vi "can_event.vi"() -> ()   [LabVIEW 2009]
doc: "This example demonstrates the use of Local Variables with Boolean controls. It uses a typical parallel loop architecture; in order to stop both loops at the same time it uses a local variable to read the switch value.\n\nThe example simulates the \"latch when pressed\" mechanical action by using another local variable to reset the switch to the FALSE value. This is needed because the actual \"latch when pressed\" mechanical action is not compatible with local variables.\n\nRefer to the \"Stopping Parallel While Loops without Reset\" example for a demonstration of what would happen if the switch was not reset."
panel:
  out "Write Error out":errorcluster {"code" format="%.0x"}
  out "Read Error out":errorcluster {"code" format="%.0x"}
  out "send status":bool
  out "receive status":bool
  out "Received MSG":string[][](table)
  in  "Receive Data Format":enum32{"Hexadecimal", "Decimal"}(radio)
  in  "MSG_RTR":bool
  in  "Flags":u8(ring)=4 items=["MSG_STD"=0, "MSG_EXT"=4]
  in  "ID (HEX)":u32=2047 format="%x"
  in  "Number to Write":u32=100
  out "Transmission MSG":string[][](table)
  in  "Write Data Format":enum32{"Hexadecimal", "Decimal"}(radio)
  in  "Read CANPort":string(combo)="CAN1"
  in  "Write CANPort":string(combo)="CAN2"
  out "GetEventMask":u32(ring)=129 items=["EV_ERR+EV_RXCHAR"=129]
  in  "ReadCount":u32=100
  out "WaitEvent\nErrorCode":u32
  in  "stop":bool
  out "Write Overlapped":T1
  out "Write Handle":u32
  out "Read Overlapped":T2
  out "Read Handle":u32
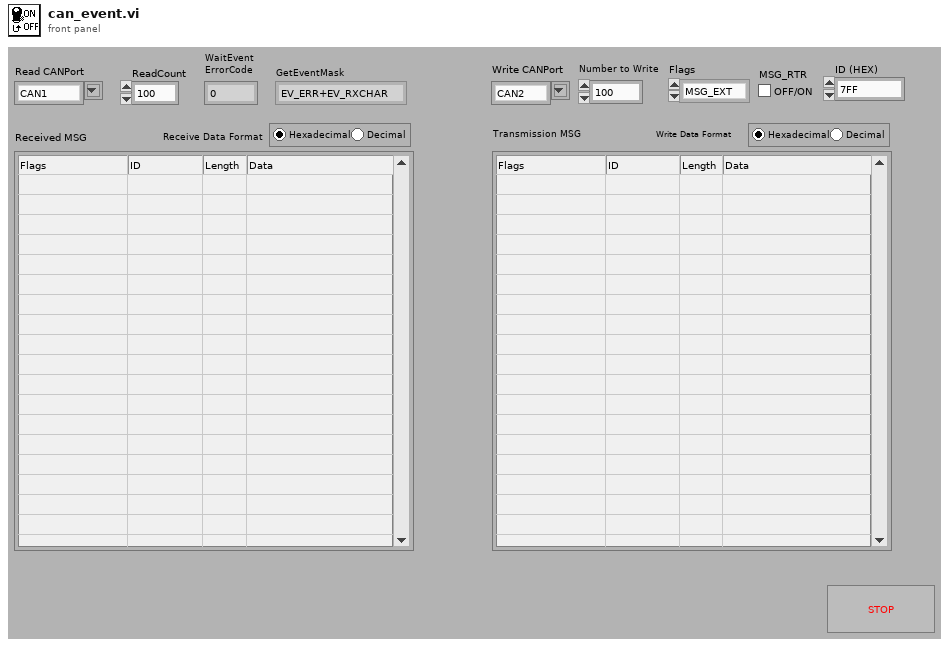
[diagram p1: front panel]
types:
  T1 = cluster{"Internal":u32, "InternalHigh":u32, "Offset":u32, "OffsetHigh":u32, "hEvent":u32}
  T2 = cluster{"Numeric":u32, "Numeric 2":u32, "Numeric 3":u32, "Numeric 4":u32, "Numeric 5":u32}
  T3 = cluster{"Flags":u32, "ID(HEX)":u32, "Length":i16, "Data":u8[]}[]
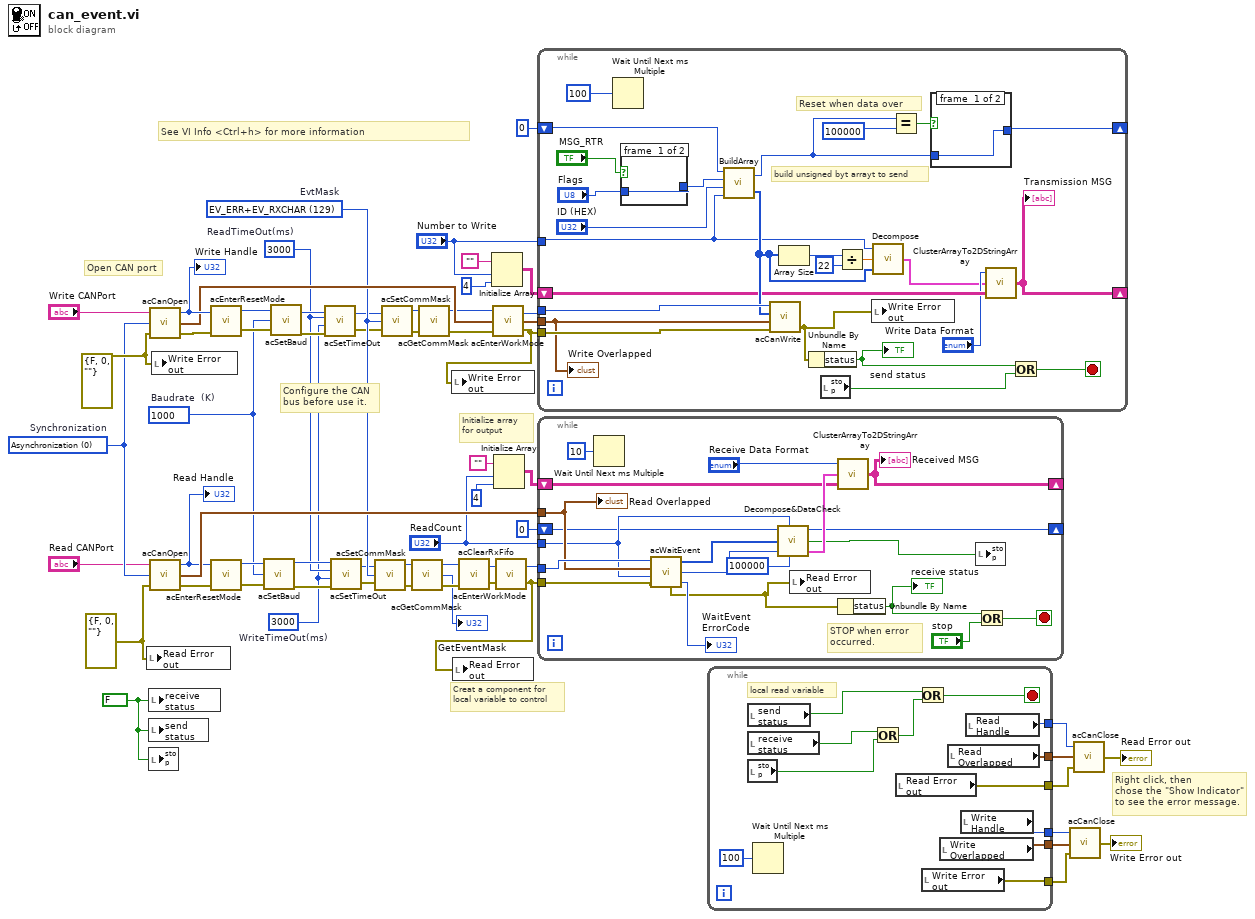
[diagram p0: block diagram]
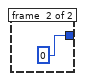
[diagram p2: hidden frame]
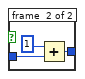
[diagram p3: hidden frame]
diagram:
  w1 = FALSE ("receive status")
  w20 = u32 3000  # WriteTimeOut(ms)
  w21 = u32 3000  # ReadTimeOut(ms)
  w19 = u16 1000 items=["10"=10, "20"=20, "50"=50, "100"=100, "125"=125, "250"=250, "500"=500, "800"=800, "1000"=1000]  # Baudrate  (K)
  w44 = 0 items=["Synchronization"=1, "Asynchronization"=0]  # Synchronization
  w45 = errorcluster {"status"=FALSE, "code"=0, "source"=""} ("Error in")
  w37 = u32 129 items=["EV_ERR+EV_RXCHAR"=129]  # EvtMask
  w54 = errorcluster {"status"=FALSE, "code"=0, "source"=""} ("Error in")
  # "Open CAN port"
  # "Creat a component for \nlocal variable to control"
  # "Configure the CAN \nbus before use it."
  # "See VI Info <Ctrl+h> for more information"
  # "Initialize array \nfor output"
  # "Right click, then \nchose the \"Show Indicator\" \nto see the error message."
  n1 = local write "Read Error out"(w54) -> ()
  n2 = local write "receive status"(w1) -> ()
  n3 = local write "send status"(w1) -> ()
  n4 = local write "stop"(w1) -> ()
  n5 = call "acCanOpen.vi"("Error in"=w45, "Synchronization"=w44, "CANPort"="Write CANPort") -> ("Error out"=w43:errorcluster, "Overlapped"=w40:T1, "Handle"=w42:u32)
  "Write Handle" <- w42
  n6 = call "acCanOpen.vi"("Error in"=w54, "Synchronization"=w44, "CANPort"="Read CANPort") -> ("Error out"=w33:errorcluster, "Overlapped"=w59:T1, "Handle"=w34:u32)
  "Read Handle" <- w34
  n7 = local write "Write Error out"(w45) -> ()
  n8 = call "acEnterResetMode.vi"("Error in"=w43, "Handle  in"=w42) -> ("Error out"=w32:errorcluster, "Handle out"=w18:u32)
  n9 = call "acEnterResetMode.vi"("Error in"=w33, "Handle  in"=w34) -> ("Error out"=w22:errorcluster, "Handle out"=w23:u32)
  n10 = call "acSetBaud.vi"("Error in"=w22, "Baudrate"=w19, "Handle  in"=w23) -> ("Error out"=w27:errorcluster, "Handle out"=w26:u32)
  n11 = call "acSetBaud.vi"("Error in"=w32, "Baudrate"=w19, "Handle  in"=w18) -> ("Error out"=w30:errorcluster, "Handle out"=w31:u32)
  n12 = call "acSetTimeOut.vi"("Error in"=w30, "WriteTimeOut"=w20, "Read TimeOut"=w21, "Handle  in"=w31) -> ("Error out"=w28:errorcluster, "Handle out"=w29:u32)
  n13 = call "acSetTimeOut.vi"("Error in"=w27, "WriteTimeOut"=w20, "Read TimeOut"=w21, "Handle  in"=w26) -> ("Error out"=w25:errorcluster, "Handle out"=w24:u32)
  n14 = call "acSetCommMask.vi"("Error in"=w25, "EventMask"=w37, "Handle  in"=w24) -> ("Error out"=w61:errorcluster, "Handle out"=w60:u32)  [unwired: 1 in]
  n15 = call "acSetCommMask.vi"("Error in"=w28, "EventMask"=w37, "Handle  in"=w29) -> ("Error out"=w39:errorcluster, "Handle out"=w38:u32)  [unwired: 1 in]
  n16 = call "acGetCommMask.vi"("Handle  in"=w60, "Error in"=w61) -> ("Handle out"=w46:u32, "GetEventMask"=→"GetEventMask":u32, "Error out"=w47:errorcluster)
  n17 = call "acGetCommMask.vi"("Handle  in"=w38, "Error in"=w39) -> ("Handle out"=w2:u32, "Error out"=w3:errorcluster)  [unwired: 1 out]
  n18 = call "acClearRxFifo.vi"("Error in"=w47, "Handle  in"=w46) -> ("Error out"=w49:errorcluster, "Handle out"=w48:u32)
  n19 = Initialize Array("", "Number to Write", 4 ("Dimension Size")) -> (w13:string[][])
  n20 = call "acEnterWorkMode.vi"("Error in"=w3, "Handle  in"=w2) -> ("Error out"=w4:errorcluster, "Handle out"=w41:u32)
  n21 = local write "Write Error out"(w4) -> ()
  n22 = Initialize Array("", "ReadCount", 4 ("Dimension Size")) -> (w8:string[][])
  n23 = call "acEnterWorkMode.vi"("Error in"=w49, "Handle  in"=w48) -> ("Error out"=w6:errorcluster, "Handle out"=w56:u32)
  n24 = local write "Read Error out"(w6) -> ()
  n25 = while {
    tunnel: w41 -> [w87]
    tunnel: w4 -> [w86]
    tunnel: w40 -> [w85]
    shift-right: [w66] -> _
    shift-left: 0 ("Numberto out") -> [w82]
    shift-right: [w75] -> _
    shift-left: w13 -> [w76]
    tunnel: "Number to Write" -> [w77]
    stop <- w62 stop-if-true
    # "Reset when data over"
    # "build unsigned byt arrayt to send"
    n26 = Wait Until Next ms Multiple(millisecond multiple=u32 100) -> ()  [unwired: 1 out]
    n27 = case shown="False" "MSG_RTR" {
      tunnel: "Flags" -> [w90 w93]
      tunnel: [w90 w91] -> w80
      frame #0 {
      }
      frame #1 {
        n28 = Add(x=u8 1, y=w93) -> (x+y=w91:u8)
      }
    }
    n29 = call "BuildArray.vi"("Number to Write"=w77, "ID"="ID (HEX)", "Flags"=w80, "Numberto in"=w82) -> ("initialized array"=w78:u8[], "Numberto out"=w67:i32)
    n30 = call "acCanWrite.vi"("Error in"=w86, "Overlapped"=w85, "MSG"=w78, "Handle  in"=w87) -> ("Error out"=w63:errorcluster)  [unwired: 2 out]
    n31 = Array Size(array=w78) -> (size(s)=w71:i32)
    n32 = Unbundle By Name(w63) -> ("status"=w64:bool)
    "send status" <- w64
    n33 = local read "stop"() -> (w65:bool)
    n34 = Divide(x=w71, y=22) -> (x/y=w72:dbl)
    n35 = local write "Write Error out"(w63) -> ()
    n36 = call "Decompose.vi"("Array"=w78, "Real"=w72, "Expect"=w77) -> ("MSG"=w70:T3)
    n37 = Equal?(x=w67, y=u32 100000) -> (x = y?=w68:bool)
    n38 = case shown="False" w68 {
      tunnel: w67 -> [w88 _]
      tunnel: [w88 u32 0 ("Numberto out")] -> w66
      frame #0 {
      }
      frame #1 {
      }
    }
    n39 = call "ClusterArrayTo2DStringArray.vi"("Input Array"=w76, "MSG"=w70, "Data Format"="Write Data Format") -> ("Output Array"=w75:string[][])
    "Transmission MSG" <- w75
    n40 = Or(x=w64, y=w65) -> (x .or. y?=w62:bool)
    "Write Overlapped" <- w85
  }
  n41 = while {
    tunnel: w56 -> [w112]
    tunnel: w6 -> [w113]
    tunnel: w59 -> [w110]
    tunnel: "ReadCount" -> [w105]
    shift-right: [w101] -> _
    shift-left: w8 -> [w104]
    shift-right: [w100] -> _
    shift-left: u32 0 ("Number to out") -> [w103]
    stop <- w94 stop-if-true
    # "STOP when error\noccurred."
    n42 = Wait Until Next ms Multiple(millisecond multiple=u32 10) -> ()  [unwired: 1 out]
    n43 = call "acWaitEvent.vi"("Error in"=w113, "ReadCount"=w105, "Overlapped"=w110, "Handle  in"=w112) -> ("ErrorCode"=→"WaitEvent\nErrorCode":u32, "Error out"=w96:errorcluster, "NumberOfRead"=w102:u32, "MSG"=w109:u8[])  [unwired: 1 out]
    n44 = call "Decompose&DataCheck.vi"("Number to in"=w103, "NumbertoRead"=w105, "Array"=w109, "NumberofRead"=w102, "threshold"=u32 100000) -> ("Number to out"=w100:u32, "check error"=w95:bool, "MSG"=w106:T3)
    n45 = local write "Read Error out"(w96) -> ()
    n46 = call "ClusterArrayTo2DStringArray.vi"("Input Array"=w104, "MSG"=w106, "Data Format"="Receive Data Format") -> ("Output Array"=w101:string[][])
    "Received MSG" <- w101
    n47 = Unbundle By Name(w96) -> ("status"=w97:bool)
    "receive status" <- w97
    n48 = local write "stop"(w95) -> ()
    n49 = Or(x=w97, y="stop") -> (x .or. y?=w94:bool)
    "Read Overlapped" <- w110
  }
  n50 = while {
    tunnel: [w125] -> w57
    tunnel: [w124] -> w55
    tunnel: [w123] -> w51
    tunnel: [w114] -> w50
    tunnel: [w122] -> w17
    tunnel: [w115] -> w5
    stop <- w117 stop-if-true
    # "local read variable"
    n51 = local read "send status"() -> (w118:bool)
    n52 = local read "receive status"() -> (w119:bool)
    n53 = local read "stop"() -> (w120:bool)
    n54 = Wait Until Next ms Multiple(millisecond multiple=u32 100) -> ()  [unwired: 1 out]
    n55 = Or(x=w119, y=w120) -> (x .or. y?=w116:bool)
    n56 = local read "Read Error out"() -> (w115:errorcluster)
    n57 = Or(x=w118, y=w116) -> (x .or. y?=w117:bool)
    n58 = local read "Write Error out"() -> (w114:errorcluster)
    n59 = local read "Write Overlapped"() -> (w122:T1)
    n60 = local read "Read Overlapped"() -> (w124:T2)
    n61 = local read "Write Handle"() -> (w123:u32)
    n62 = local read "Read Handle"() -> (w125:u32)
  }
  n63 = call "acCanClose.vi"("Error in"=w50, "Overlapped"=w17, "Handle  in"=w51) -> ("Error out"=→"Write Error out":errorcluster)
  n64 = call "acCanClose.vi"("Error in"=w5, "Overlapped"=w55, "Handle  in"=w57) -> ("Error out"=→"Read Error out":errorcluster)
